vi "Begin.vi"(8 "error in":errorcluster) -> (0 "error out":errorcluster)   [LabVIEW 2015]
doc: "Called before other user functions, this VI is expected to open initial I/O refnums, load in file data, and do all program initialization. Notice that the <B>error out</B> terminal is simply used for data flow. Wiring it to other structures or subVIs ensures that this VI runs first."
uses:
  <vilib>/Rock Robotics/SystemInterfaces/spilib/spi_bus.ctl
  <vilib>/Rock Robotics/WPI/Accelerometer/ADXL362 Range.ctl
  <vilib>/Rock Robotics/WPI/Accelerometer/WPI_AccelerometerADXL345 Axes.ctl
  <vilib>/Rock Robotics/SystemInterfaces/DIO/FPGA_DIOPWMChannel.ctl
  <vilib>/Rock Robotics/WPI/SafetyOutput/WPI_SafetyOutputConfigMenu.ctl
  <vilib>/Rock Robotics/WPI/DriverStation/WPI_DriverStationRobotMode2.ctl
  <vilib>/Rock Robotics/WPI/Joystick/WPI_JoystickDeviceEnum.ctl
  <vilib>/Rock Robotics/SystemInterfaces/DIO/FPGA_DIOChannel.ctl
  <vilib>/Rock Robotics/WPI/RobotDrive/WPI_RobotDriveOpen2MotorWithTalon.vi
  Robot Global Data.vi
  <vilib>/Rock Robotics/Network Tables/NT Write String Array.vi
  <vilib>/Rock Robotics/WPI/Solenoid/WPI_SolenoidOpenSingle.vi
  <vilib>/Rock Robotics/WPI/Counter/WPI_CounterDigitalInputToDigitalSource.vi
  <vilib>/Rock Robotics/WPI/MotorControl/WPI_MotorControlOpen VictorSP.vi
  <vilib>/Rock Robotics/WPI/Gyro/WPI_GyroAnalogOpen.vi
  <vilib>/Rock Robotics/WPI/Gyro/WPI_GyroXRS450_SPI_Open.vi
  <vilib>/Rock Robotics/WPI/Accelerometer/WPI_AccelerometerADXL362_SPI_Open.vi
panel:
  in  "ADXL345 Axes":T1={"X-Axis"=TRUE, "Y-Axis"=FALSE, "Z-Axis"=FALSE}
  in  "SPI Bus":T2=enum."SPI On-Board, CS1"
  in  "Accel Range":T3 items=["+/- 2 g", "+/- 4 g", "+/- 8 g"]
  in  "SPI Bus 2":T2
  in  "Sample Rate (ms)":dbl=1.0 min=0.0 max=100.0 step=0.25 format="%#_13g"
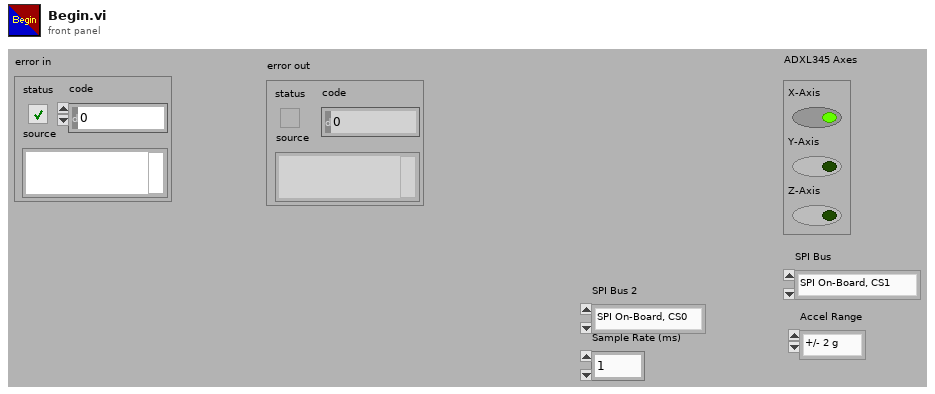
[diagram p1: front panel]
types:
  T1 = typedef "WPI_AccelerometerADXL345 Axes.ctl" = cluster{"X-Axis":bool, "Y-Axis":bool, "Z-Axis":bool}
  T2 = typedef "spi_bus.ctl" = enum16{"SPI On-Board, CS0", "SPI On-Board, CS1", "SPI On-Board, CS2", "SPI On-Board, CS3", "SPI MXP", "Invalid"}
  T3 = typedef "ADXL362 Range.ctl" = u8
  T4 = typedef "FPGA_DIOChannel.ctl" = enum8{"DIO 0", "DIO 1", "DIO 2", "DIO 3", "DIO 4", "DIO 5", "DIO 6", "DIO 7", "DIO 8", "DIO 9", "DIO MXP 0", "DIO MXP 1", "DIO MXP 2", "DIO MXP 3", "DIO MXP 4", "DIO MXP 5", "DIO MXP 6", "DIO MXP 7", "DIO MXP 8", "DIO MXP 9", "DIO MXP 10", "DIO MXP 11", "DIO MXP 12", "DIO MXP 13", "DIO MXP 14", "DIO MXP 15", "Invalid"}
  T5 = enum16{"Relay 0", "Relay 1", "Relay 2", "Relay 3"}
  T6 = typedef "FPGA_DIOPWMChannel.ctl" = enum8{"PWM 0", "PWM 1", "PWM 2", "PWM 3", "PWM 4", "PWM 5", "PWM 6", "PWM 7", "PWM 8", "PWM 9", "PWM MXP 0", "PWM MXP 1", "PWM MXP 2", "PWM MXP 3", "PWM MXP 4", "PWM MXP 5", "PWM MXP 6", "PWM MXP 7", "PWM MXP 8", "PWM MXP 9", "Invalid"}
  T7 = typedef "WPI_JoystickDeviceEnum.ctl" = enum16{"USB 0", "USB 1", "USB 2", "USB 3", "USB 4", "USB 5"}
  T8 = enum16{"Solenoid 0", "Solenoid 1", "Solenoid 2", "Solenoid 3", "Solenoid 4", "Solenoid 5", "Solenoid 6", "Solenoid 7"}
  T9 = typedef "WPI_DriverStationRobotMode2.ctl" = enum16{"Autonomous Disabled", "Autonomous Enabled", "Teleop Disabled", "Teleop Enabled", "Disconnected", "Finish", "Test Disabled", "Test Enabled", "Emergency Stopped"}
  T10 = typedef "WPI_SafetyOutputConfigMenu.ctl" = enum16{"Enable", "Disable"}
  T11 = typedef "WPI_JoystickDevRef.ctl" = cluster{"Device":T7}
  T12 = typedef "WPI_DigitalInputDevRef.ctl" = cluster{"DevStatus":errorcluster, "DIO Channel":T4}
  T13 = typedef "WPI_SolenoidDevRef.ctl" = cluster{"DevStatus":errorcluster, "Pneumatics Control Module":u8, "Forward Solenoid Channel":T14, "Reverse Solenoid Channel":T14}
  T14 = typedef "WPI_SolenoidChannel.ctl" = enum8{"Solenoid 0", "Solenoid 1", "Solenoid 2", "Solenoid 3", "Solenoid 4", "Solenoid 5", "Solenoid 6", "Solenoid 7", "Invalid"}
  T15 = typedef "WPI_MotorControlDeviceRef.ctl" = cluster{"DeviceStatus":errorcluster, "Type":T16, "PWM":cluster{"PWM Channel":T6, "DeadBand":T17}, "CAN":cluster{"Device Number":u8, "Control Mode":T18, "Semaphore":T19, "Max Vout":dbl, "TalonSRX Control Mode":T20}, "Invert":bool}
  T16 = typedef "WPI_MotorControlType.ctl" = enum16{"PWM", "CAN", "CANTalonSRX"}
  T17 = typedef "WPI_PWMDeadband.ctl" = cluster{"Name":string, "maxPositivePwm":i32, "minPositivePwm":i32, "centerPwm":i32, "maxNegativePwm":i32, "minNegativePwm":i32, "angularRange":u16}
  T18 = typedef "WPI_CANJaguar_ControlMode.ctl" = enum8{"Percent VBus", "Current", "Speed", "Position", "Voltage"}
  T19 = typedef "Semaphore RefNum" = refnum<k1>
  T20 = typedef "WPI_CANTalonSRX_APIControlMode.ctl" = enum8{"Percent VBus", "Speed", "Position", "Slave", "Unchanged / Invalid", "Voltage Compensation", "Current", "Motion Profile"}
  T21 = typedef "FPGA_CounterEncoderSourceConvertionLVSourceType.ctl" = cluster{"DevStatus":errorcluster, "AnalogTriggerMode?":bool, "DigitalMode":cluster{"DIO Channel":T22}, "AnalogTriggerMode":cluster{"AnalogTriggerIndex":T23, "OutputType":T24}}
  T22 = typedef "FPGA_DIODigitalSourceChannel.ctl" = enum8{"DIO 0", "DIO 1", "DIO 2", "DIO 3", "DIO 4", "DIO 5", "DIO 6", "DIO 7", "DIO 8", "DIO 9", "DIO MXP 0", "DIO MXP 1", "DIO MXP 2", "DIO MXP 3", "DIO MXP 4", "DIO MXP 5", "DIO MXP 6", "DIO MXP 7", "DIO MXP 8", "DIO MXP 9", "DIO MXP 10", "DIO MXP 11", "DIO MXP 12", "DIO MXP 13", "DIO MXP 14", "DIO MXP 15", "Disabled"}
  T23 = typedef "FPGA_AnalogTriggerIndex.ctl" = enum8{"Trig 0", "Trig 1", "Trig 2", "Trig 3", "Trig 4", "Trig 5", "Trig 6", "Trig 7", "Invalid"}
  T24 = typedef "FPGA_AnalogTriggerOutType.ctl" = enum16{"InWindow", "TriggerState", "Rising", "Falling"}
  T25 = typedef "WPI_RobotDriveDevRef.ctl" = cluster{"DevStatus":errorcluster, "Motors[]":T15[], "Square Inputs":bool, "Max Output":dbl}
  T26 = typedef "WPI_RelayDevRef.ctl" = cluster{"DevStatus":errorcluster, "Relay Channel":T27, "Relay Direction":T28}
  T27 = typedef "FPGA_DIORelayChannel.ctl" = enum8{"Relay 0", "Relay 1", "Relay 2", "Relay 3", "Invalid"}
  T28 = typedef "WPI_RelayDirection.ctl" = enum16{"Both directions", "Forward only", "Reverse only"}
  T29 = typedef "WPI_PotentiometerDevRef.ctl" = cluster{"DevStatus":errorcluster, "Analog Channel":T30, "Invert Output":bool}
  T30 = typedef "FPGA_AIChannel.ctl" = enum8{"AI 0", "AI 1", "AI 2", "AI 3", "AI MXP 0", "AI MXP 1", "AI MXP 2", "AI MXP 3", "Invalid"}
  T31 = typedef "WPI_EncoderDevRef.ctl" = cluster{"DevStatus":errorcluster, "EncoderIndex":T32, "CounterIndex":T33, "DistancePerCount":dbl, "Decoding Type":T34}
  T32 = typedef "FPGA_EncoderIdx.ctl" = enum8{"Enc 0", "Enc 1", "Enc 2", "Enc 3", "Enc 4", "Enc 5", "Enc 6", "Enc 7", "Invalid"}
  T33 = typedef "FPGA_CounterCtrSystemIndex.ctl" = enum8{"Ctr 0", "Ctr 1", "Ctr 2", "Ctr 3", "Ctr 4", "Ctr 5", "Ctr 6", "Ctr 7", "Invalid"}
  T34 = typedef "WPI_EncoderType.ctl" = enum16{"1x", "2x", "4x"}
  T35 = typedef "WPI_ServoDeviceRef.ctl" = cluster{"DeviceStatus":errorcluster, "PWM Channel":T6, "DeadBand":T17}
  T36 = typedef "WPI_GyroDevRef.ctl" = cluster{"DevStatus":errorcluster, "Analog Channel":T30, "Offset":dbl, "Gain (VoltsPerDegree/Second)":dbl, "Gyro Type":enum16{"Analog", "XRS450"}, "Handle":i32, "SPI Bus":T2, "Device Found":bool, "Sample Rate":dbl, "Calibrate On Open":bool}
  T37 = typedef "WPI_AccelerometerDevRef.ctl" = cluster{"DevStatus":errorcluster, "Scaling":T38, "Analog Channels":T39, "I2C Bus":T40, "SPI Bus":T2, "Accel Range":T41, "ADXL Axes":T1, "Handle":i32, "Device Address":u8, "Accel Type":enum16{"Analog", "ADXL345 I2C", "ADXL345 SPI", "Internal", "ADXL362 SPI"}}
  T38 = typedef "WPI_AccelerometerScaling.ctl" = cluster{"Gain (VoltsPerG)":dbl, "Center Voltage":dbl}
  T39 = typedef "WPI_AccelerometerAnalogChannels.ctl" = cluster{"X-Axis":T30, "Y-Axis":T30, "Z-Axis":T30}
  T40 = typedef "i2c_bus.ctl" = enum16{"I2C On-Board", "I2C MXP", "Invalid"}
  T41 = typedef "ADXL345 Range.ctl" = u8
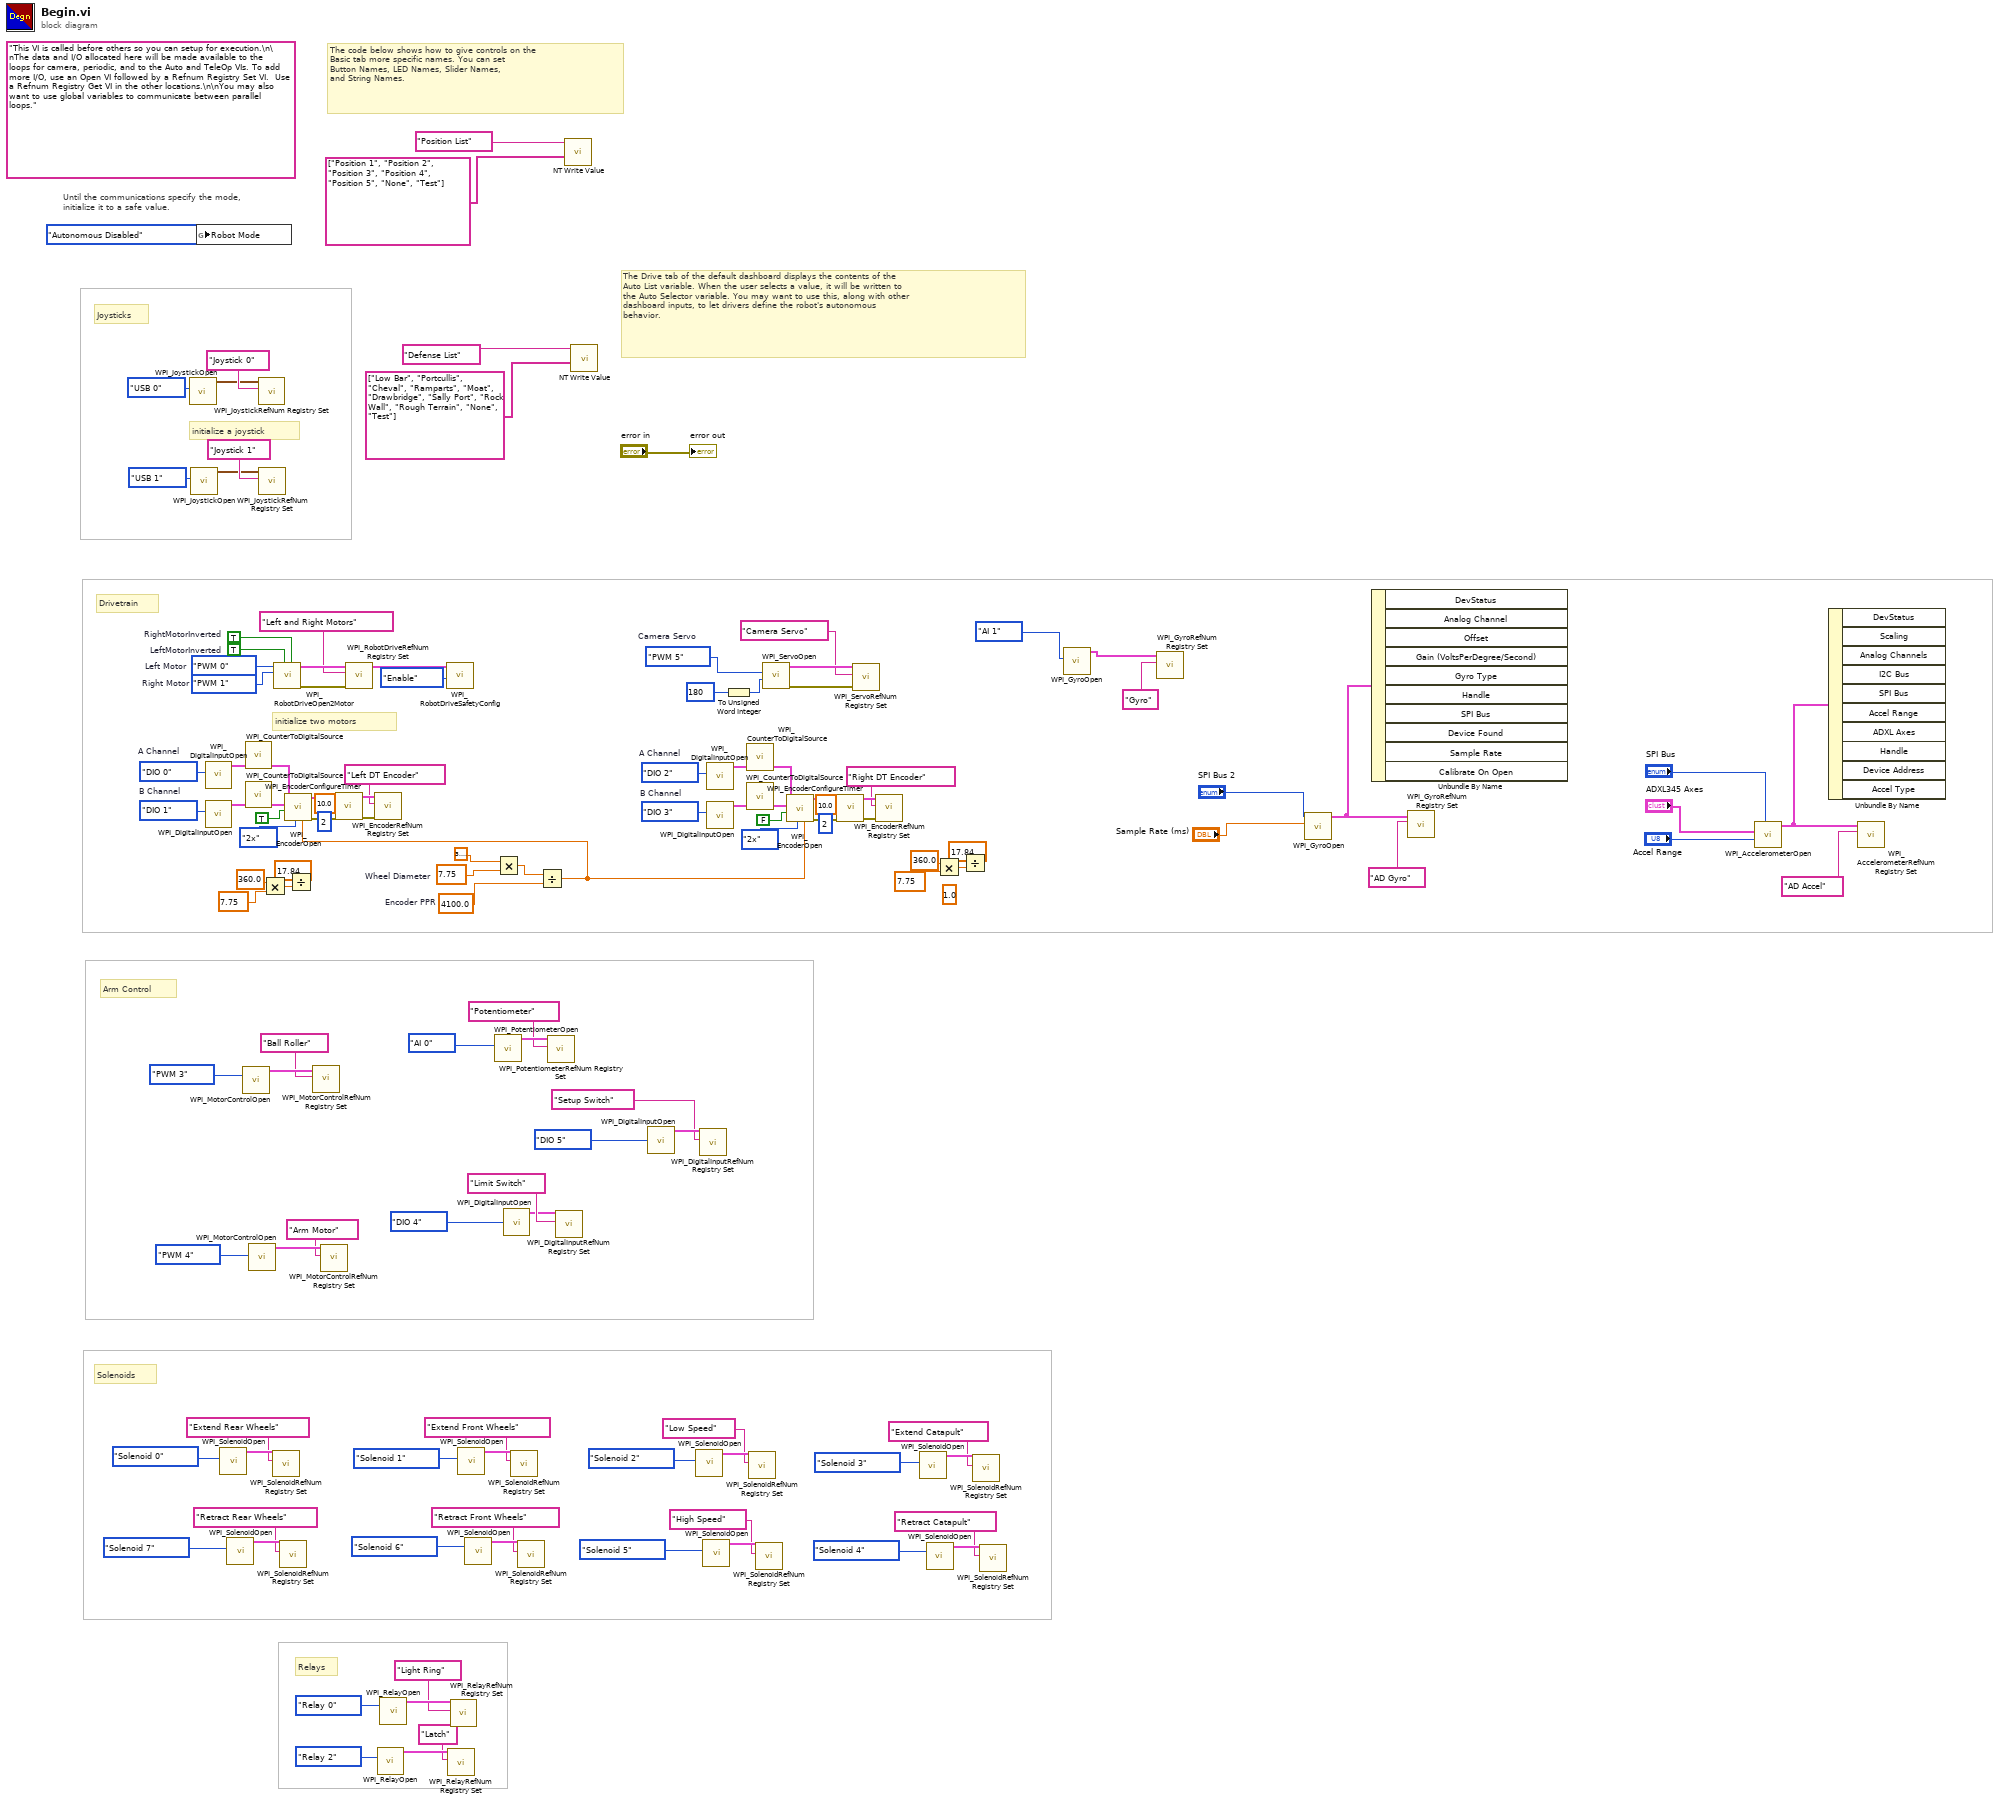
[diagram p0: block diagram]
diagram:
  (unwired) 1.0
  w18 = 4100.0  # Encoder PPR
  w19 = 7.75  # Wheel Diameter
  w31 = FPGA_DIOPWMChannel."PWM 5"  # Camera Servo
  w52 = FPGA_DIOChannel."DIO 3"  # B Channel
  w51 = FPGA_DIOChannel."DIO 2"  # A Channel
  w80 = FPGA_DIOChannel."DIO 1"  # B Channel
  w79 = FPGA_DIOChannel."DIO 0"  # A Channel
  (unwired) "This VI is called before others so you can setup for execution.\n\nThe data and I/O allocated here will be made available to the loops for camera, periodic, and to the Auto and TeleOp VIs. To add more I/O, use an Open VI followed by a Refnum Registry Set VI.  Use a Refnum Registry Get VI in the other locations.\n\nYou may also want to use global variables to communicate between parallel loops."
  w121 = FPGA_DIOPWMChannel."PWM 1"  # Right Motor
  w122 = FPGA_DIOPWMChannel."PWM 0"  # Left Motor
  w126 = TRUE  # LeftMotorInverted
  w127 = TRUE  # RightMotorInverted
  # "Relays"
  # "Drivetrain"
  # "Arm Control"
  # "Joysticks"
  # "Solenoids"
  # "The Drive tab of the default dashboard displays the contents of the\nAuto List variable. When the user selects a value, it will be written to\nthe Auto Selector variable. You may want to use this, along with other\ndashboard inputs, to let drivers define the robot's autonomous\nbehavior."
  # "The code below shows how to give controls on the\nBasic tab more specific names. You can set\nButton Names, LED Names, Slider Names,\nand String Names."
  # "initialize a joystick"
  # "Until the communications specify the mode,\ninitialize it to a safe value."
  # "initialize two motors"
  n1 = call <vilib>:"WPI_JoystickOpen.vi"("JoystickDevice"=WPI_JoystickDeviceEnum."USB 0") -> ("JoystickDevRef"=w116:T11)  [unwired: 10 in]
  n2 = call <vilib>:"WPI_JoystickOpen.vi"("JoystickDevice"=WPI_JoystickDeviceEnum."USB 1") -> ("JoystickDevRef"=w84:T11)  [unwired: 10 in]
  n3 = global write "Robot Global Data.vi" "Robot Mode"(WPI_DriverStationRobotMode2."Autonomous Disabled" ("Robot Mode")) -> ()
  n4 = call <vilib>:"WPI_DigitalInputOpen.vi"("DIO Channel"=w79) -> ("DigitalInputDevRef"=w76:T12)  [unwired: 1 in, 9 out]
  n5 = call <vilib>:"WPI_DigitalInputOpen.vi"("DIO Channel"=w80) -> ("DigitalInputDevRef"=w77:T12)  [unwired: 1 in, 9 out]
  n6 = call-poly <vilib>:"WPI_SolenoidOpen.vi"("Solenoid Channel"=T8."Solenoid 0") -> ("SolenoidDevRef"=w107:T13)  [unwired: 9 in, 1 out]
  n7 = call-poly <vilib>:"WPI_SolenoidOpen.vi"("Solenoid Channel"=T8."Solenoid 7") -> ("SolenoidDevRef"=w109:T13)  [unwired: 9 in, 1 out]
  n8 = call-poly <vilib>:"WPI_MotorControlOpen.vi"("PWM Channel"=FPGA_DIOPWMChannel."PWM 3") -> ("MotorControlDeviceRef"=w60:T15)  [unwired: 9 in, 1 out]
  n9 = call-poly <vilib>:"WPI_CounterToDigitalSource.vi"("DigitalInputDevRef"=w76) -> ("Digital Source"=w75:T21)  [unwired: 6 out]
  n10 = call-poly <vilib>:"WPI_CounterToDigitalSource.vi"("DigitalInputDevRef"=w77) -> ("Digital Source"=w78:T21)  [unwired: 6 out]
  n11 = call-poly <vilib>:"WPI_MotorControlOpen.vi"("PWM Channel"=FPGA_DIOPWMChannel."PWM 4") -> ("MotorControlDeviceRef"=w55:T15)  [unwired: 9 in, 1 out]
  n12 = call <vilib>:"WPI_JoystickRefNum Registry Set.vi"("refnum name"="Joystick 0", "JoystickDevRef"=w116) -> ()  [unwired: 8 in, 2 out]
  n13 = call <vilib>:"WPI_JoystickRefNum Registry Set.vi"("refnum name"="Joystick 1", "JoystickDevRef"=w84) -> ()  [unwired: 8 in, 2 out]
  n14 = Multiply(x=360.0, y=7.75) -> (x*y=w66:dbl)
  n15 = call <vilib>:"WPI_SolenoidRefNum Registry Set.vi"("refnum name"="Extend Rear Wheels", "SolenoidDevRef"=w107) -> ()  [unwired: 8 in, 2 out]
  n16 = call-poly <vilib>:"WPI_RobotDriveOpen2Motor.vi"("Right Motor Inverted"=w127, "Left Motor Inverted"=w126, "Right Motor"=w121, "Left Motor"=w122) -> ("error out"=w123:errorcluster, "RobotDriveDevRef"=w125:T25)  [unwired: 1 in, 5 out]
  n17 = call <vilib>:"WPI_SolenoidRefNum Registry Set.vi"("refnum name"="Retract Rear Wheels", "SolenoidDevRef"=w109) -> ()  [unwired: 8 in, 2 out]
  n18 = Divide(x=17.84, y=w66) -> ()  [unwired: 1 out]
  n19 = call <vilib>:"WPI_MotorControlRefNum Registry Set.vi"("refnum name"="Ball Roller", "MotorControlDevRef"=w60) -> ()  [unwired: 8 in, 2 out]
  n20 = call <vilib>:"WPI_MotorControlRefNum Registry Set.vi"("refnum name"="Arm Motor", "MotorControlDevRef"=w55) -> ()  [unwired: 8 in, 2 out]
  n21 = call <vilib>:"WPI_RobotDriveRefNum Registry Set.vi"("error in (no error)"=w123, "refnum name"="Left and Right Motors", "RobotDriveDevRef"=w125) -> ("RobotDriveDevRef"=w120:T25)  [unwired: 1 in, 7 out]
  n22 = call <vilib>:"WPI_RelayOpen.vi"("Relay Channel"=T5."Relay 2") -> ("RelayDevRef"=w24:T26)  [unwired: 9 in, 1 out]
  n23 = call <vilib>:"WPI_RelayOpen.vi"("Relay Channel"=T5."Relay 0") -> ("RelayDevRef"=w27:T26)  [unwired: 9 in, 1 out]
  n24 = call <vilib>:"WPI_RobotDriveSafetyConfig.vi"("mode"=WPI_SafetyOutputConfigMenu."Enable", "RobotDriveDevRef"=w120) -> ()  [unwired: 8 in, 2 out]
  n25 = call <vilib>:"WPI_RelayRefNum Registry Set.vi"("refnum name"="Latch", "RelayDevRef"=w24) -> ()  [unwired: 8 in, 2 out]
  n26 = call <vilib>:"WPI_RelayRefNum Registry Set.vi"("refnum name"="Light Ring", "RelayDevRef"=w27) -> ()  [unwired: 8 in, 2 out]
  n27 = call-poly <vilib>:"WPI_SolenoidOpen.vi"("Solenoid Channel"=T8."Solenoid 1") -> ("SolenoidDevRef"=w101:T13)  [unwired: 9 in, 1 out]
  n28 = call-poly <vilib>:"WPI_SolenoidOpen.vi"("Solenoid Channel"=T8."Solenoid 6") -> ("SolenoidDevRef"=w103:T13)  [unwired: 9 in, 1 out]
  n29 = call <vilib>:"WPI_PotentiometerOpen.vi"("Analog Channel"=enum16{"AI 0"}."AI 0") -> ("PotDevRef"=w58:T29)  [unwired: 9 in, 1 out]
  n30 = Multiply(x=3.141592653589793, y=w19) -> (x*y=w17:dbl)
  n31 = call <vilib>:"WPI_DigitalInputOpen.vi"("DIO Channel"=FPGA_DIOChannel."DIO 4") -> ("DigitalInputDevRef"=w81:T12)  [unwired: 9 in, 1 out]
  n32 = call <vilib>:"WPI_SolenoidRefNum Registry Set.vi"("refnum name"="Extend Front Wheels", "SolenoidDevRef"=w101) -> ()  [unwired: 8 in, 2 out]
  n33 = call <vilib>:"WPI_SolenoidRefNum Registry Set.vi"("refnum name"="Retract Front Wheels", "SolenoidDevRef"=w103) -> ()  [unwired: 8 in, 2 out]
  n34 = Divide(x=w17, y=w18) -> (x/y=w4:dbl)
  n35 = call <vilib>:"WPI_EncoderOpen.vi"("DistancePerCount"=w4, "Decoding Type"=enum16{"1x", "2x", "4x"}."2x", "Invert Direction (False)"=TRUE, "BSource"=w78, "ASource"=w75) -> ("error out"=w74:errorcluster, "EncoderDevRef"=w73:T31)  [unwired: 3 in, 2 out]
  n36 = call <vilib>:"WPI_EncoderConfigureTimer.vi"("error in (no error)"=w74, "Number Samples to Average"=2, "Minimum Rate"=10.0, "EncoderDevRef"=w73) -> ("error out"=w72:errorcluster, "EncoderDevRef"=w71:T31)  [unwired: 6 in]
  n37 = call <vilib>:"WPI_EncoderRefNum Registry Set.vi"("error in (no error)"=w72, "refnum name"="Left DT Encoder", "EncoderDevRef"=w71) -> ()  [unwired: 7 in, 2 out]
  n38 = call <vilib>:"WPI_PotentiometerRefNum Registry Set.vi"("refnum name"="Potentiometer", "PotDevRef"=w58) -> ()  [unwired: 8 in, 2 out]
  n39 = call <vilib>:"WPI_DigitalInputRefNum Registry Set.vi"("refnum name"="Limit Switch", "DigitalInputDevRef"=w81) -> ()  [unwired: 8 in, 2 out]
  n40 = call-poly <vilib>:"NT Write Value.vi"("String Array"=string[] ["Position 1", "Position 2", "Position 3", "Position 4", "Position 5", "None", "Test"], "Name"="Position List") -> ()  [unwired: 9 in, 1 out]
  n41 = call-poly <vilib>:"NT Write Value.vi"("String Array"=string[] ["Low Bar", "Portcullis", "Cheval", "Ramparts", "Moat", "Drawbridge", "Sally Port", "Rock Wall", "Rough Terrain", "None", "Test"], "Name"="Defense List") -> ()  [unwired: 9 in, 1 out]
  n42 = call <vilib>:"WPI_DigitalInputOpen.vi"("DIO Channel"=FPGA_DIOChannel."DIO 5") -> ("DigitalInputDevRef"=w2:T12)  [unwired: 9 in, 1 out]
  n43 = call-poly <vilib>:"WPI_SolenoidOpen.vi"("Solenoid Channel"=T8."Solenoid 2") -> ("SolenoidDevRef"=w95:T13)  [unwired: 9 in, 1 out]
  n44 = call <vilib>:"WPI_DigitalInputRefNum Registry Set.vi"("refnum name"="Setup Switch", "DigitalInputDevRef"=w2) -> ()  [unwired: 8 in, 2 out]
  n45 = call-poly <vilib>:"WPI_SolenoidOpen.vi"("Solenoid Channel"=T8."Solenoid 5") -> ("SolenoidDevRef"=w97:T13)  [unwired: 9 in, 1 out]
  n46 = call <vilib>:"WPI_DigitalInputOpen.vi"("DIO Channel"=w51) -> ("DigitalInputDevRef"=w48:T12)  [unwired: 1 in, 9 out]
  n47 = call <vilib>:"WPI_DigitalInputOpen.vi"("DIO Channel"=w52) -> ("DigitalInputDevRef"=w49:T12)  [unwired: 1 in, 9 out]
  n48 = To Unsigned Word Integer(number=180) -> (unsigned 16bit integer=w5:u16)
  n49 = call-poly <vilib>:"WPI_CounterToDigitalSource.vi"("DigitalInputDevRef"=w48) -> ("Digital Source"=w47:T21)  [unwired: 6 out]
  n50 = call-poly <vilib>:"WPI_CounterToDigitalSource.vi"("DigitalInputDevRef"=w49) -> ("Digital Source"=w50:T21)  [unwired: 6 out]
  n51 = call <vilib>:"WPI_SolenoidRefNum Registry Set.vi"("refnum name"="Low Speed", "SolenoidDevRef"=w95) -> ()  [unwired: 8 in, 2 out]
  n52 = call <vilib>:"WPI_SolenoidRefNum Registry Set.vi"("refnum name"="High Speed", "SolenoidDevRef"=w97) -> ()  [unwired: 8 in, 2 out]
  n53 = call <vilib>:"WPI_ServoOpen.vi"("Angular Range"=w5, "PWM Channel"=w31) -> ("error out"=w32:errorcluster, "ServoDeviceRef"=w33:T35)  [unwired: 8 in]
  n54 = call <vilib>:"WPI_EncoderOpen.vi"("DistancePerCount"=w4, "Decoding Type"=enum16{"1x", "2x", "4x"}."2x", "Invert Direction (False)"=FALSE, "BSource"=w50, "ASource"=w47) -> ("error out"=w46:errorcluster, "EncoderDevRef"=w45:T31)  [unwired: 3 in, 2 out]
  n55 = call <vilib>:"WPI_EncoderConfigureTimer.vi"("error in (no error)"=w46, "Number Samples to Average"=2, "Minimum Rate"=10.0, "EncoderDevRef"=w45) -> ("error out"=w44:errorcluster, "EncoderDevRef"=w43:T31)  [unwired: 6 in]
  n56 = call <vilib>:"WPI_ServoRefNum Registry Set.vi"("error in (no error)"=w32, "refnum name"="Camera Servo", "ServoDeviceRef"=w33) -> ()  [unwired: 7 in, 2 out]
  n57 = call <vilib>:"WPI_EncoderRefNum Registry Set.vi"("error in (no error)"=w44, "refnum name"="Right DT Encoder", "EncoderDevRef"=w43) -> ()  [unwired: 7 in, 2 out]
  n58 = call-poly <vilib>:"WPI_SolenoidOpen.vi"("Solenoid Channel"=T8."Solenoid 3") -> ("SolenoidDevRef"=w89:T13)  [unwired: 9 in, 1 out]
  n59 = call-poly <vilib>:"WPI_SolenoidOpen.vi"("Solenoid Channel"=T8."Solenoid 4") -> ("SolenoidDevRef"=w91:T13)  [unwired: 9 in, 1 out]
  n60 = Multiply(x=360.0, y=7.75) -> (x*y=w38:dbl)
  n61 = Divide(x=17.84, y=w38) -> ()  [unwired: 1 out]
  n62 = call <vilib>:"WPI_SolenoidRefNum Registry Set.vi"("refnum name"="Extend Catapult", "SolenoidDevRef"=w89) -> ()  [unwired: 8 in, 2 out]
  n63 = call <vilib>:"WPI_SolenoidRefNum Registry Set.vi"("refnum name"="Retract Catapult", "SolenoidDevRef"=w91) -> ()  [unwired: 8 in, 2 out]
  n64 = call-poly <vilib>:"WPI_GyroOpen.vi"("Analog Channel"=enum16{"AI 0", "AI 1"}."AI 1") -> ("GyroDevRef"=w26:T36)  [unwired: 8 in, 2 out]
  n65 = call <vilib>:"WPI_GyroRefNum Registry Set.vi"("refnum name"="Gyro", "GyroDevRef"=w26) -> ()  [unwired: 8 in, 2 out]
  n66 = call-poly <vilib>:"WPI_GyroOpen.vi"("Sample Rate (ms)"="Sample Rate (ms)", "SPI Bus"="SPI Bus 2") -> ("GyroDevRef"=w12:T36)  [unwired: 8 in, 1 out]
  n67 = Unbundle By Name(w12) -> ()  [unwired: 10 out]
  n68 = call <vilib>:"WPI_GyroRefNum Registry Set.vi"("refnum name"="AD Gyro", "GyroDevRef"=w12) -> ()  [unwired: 8 in, 2 out]
  n69 = call-poly <vilib>:"WPI_AccelerometerOpen.vi"("SPI Bus"="SPI Bus", "Accel Range"="Accel Range", "ADXL345 Axes"="ADXL345 Axes") -> ("AccelerometerDevRef"=w7:T37)  [unwired: 7 in, 1 out]
  n70 = Unbundle By Name(w7) -> ()  [unwired: 10 out]
  n71 = call <vilib>:"WPI_AccelerometerRefNum Registry Set.vi"("refnum name"="AD Accel", "AccelerometerDevRef"=w7) -> ()  [unwired: 8 in, 2 out]
  "error out" <- "error in"
